vi "LabVIEW_MQTT_Toolkit_V2.vi"() -> ()   [LabVIEW 2021] (continued)
                  n338 = To Double Precision Float(number=w770) -> (double precision float=w775:dbl)
                  n339 = Number To Decimal String(number=w779) -> (decimal integer string=w778:string)  [unwired: 1 in]
                  n340 = Number To Fractional String(number=w777, precision (6)=i16 3 ("width (-)")) -> (F-format string=w781:string)  [unwired: 2 in]
                  n341 = Divide(x=w775, y=w771) -> (x/y=w776:dbl)
                  n342 = To Unsigned Quad Integer(1:w774) -> (0:w773:u64)
                  n343 = Build Array(w778, w781) -> (w780:string[])
                  n344 = call "Unix Time to Timestamp.vi"("Fractional Second"=w776, "Unix Time (s)"=w773) -> ("Timestamp"=w764:timestamp)  [unwired: 8 in, 1 out]
                  n345 = Format Date/Time String(seconds (now)=w764, UTC format=TRUE) -> (date/time string=w765:string)  [unwired: 1 in]
                  n346 = Scan From String(format string="%<%x %H:%M:%S%3u>T", input string=w765) -> (output 1=w766:timestamp)  [unwired: 3 in, 3 out]
                  n347 = To Double Precision Float(number=w766) -> (double precision float=w763:dbl)
                }
                n348 = Concatenate Strings(w724, "TimeStamp;MeasureCh_Y(g);", "\n") -> (w740:string)
                n349 = Concatenate Strings(w747, "_" ("string"), "streaming.csv") -> (w748:string)
                n350 = call <vilib>:"Get System Directory.vi"("system directory type"=w731) -> ("system directory"=w741:path)  [unwired: 10 in]
                n351 = Build Path(base path=w741, name or relative path="Logfile") -> (appended path=w742:path)
                n352 = call <vilib>:"Check if File or Folder Exists.vi"("path"=w742) -> ("file or folder exists?"=w743:bool, "dup path"=w744:path)  [unwired: 8 in, 1 out]
                n353 = case shown="False" w743 {
                  tunnel: w744 -> [w761 w762]
                  tunnel: [w760 w762] -> w745
                  frame False {
                    n354 = Create Folder(path (use dialog)=w761) -> (created path=w760:path)  [unwired: 2 in, 2 out]
                  }
                  frame True {
                  }
                }
                n355 = Build Path(base path=w745, name or relative path=w748) -> (appended path=w746:path)
                n356 = Open/Create/Replace File(file path (use dialog)=w746, operation (0:open)=T11."open or create") -> (refnum out=w739:refnum<file>, error out=w737:errorcluster)  [unwired: 4 in, 1 out]
                n357 = Write to Text File(file (use dialog)=w739, text=w740, error in=w737) -> (refnum out=w738:refnum<file>, error out=w736:errorcluster)  [unwired: 1 in, 1 out]
                n358 = Close File(refnum=w738, error in=w736) -> (path=w725:path)  [unwired: 1 out]
              }
              frame 5 {
                w790 = T14 2 items=["User Home"=0, "User Desktop"=1, "User Documents"=2, "User Application Data"=3, "User Preferences"=4, "User Temporary"=5, "Public Documents"=6, "Public Application Data"=7, "Public Preferences"=8, "Public Cache"=13, "System Core Libraries"=9, "System Installed Libraries"=10, "Application Files"=11, "Boot Volume Root"=12] ("system directory type")
                n359 = Decimate 1D Array(w820) -> (w816:dbl[], w817:dbl[])
                n360 = Search and Replace String(replace all?=TRUE ("replace all? (F)"), input string=w784, search string="/") -> (result string=w806:string)  [unwired: 5 in, 3 out]
                n361 = Concatenate Strings(w783, "TimeStamp;MeasureCh_Z(g);Ch_Y(g);", "\n") -> (w799:string)
                n362 = for {
                  tunnel: [w843] -> w818 mode=indexing
                  tunnel: w819 -> [w842] mode=indexing
                  tunnel: w816 -> [w840] mode=indexing
                  tunnel: w817 -> [w839] mode=indexing
                  tunnel: [w840] -> w815 mode=indexing
                  tunnel: [w839] -> w814 mode=indexing
                  tunnel: w813 -> [w834]
                  tunnel: w812 -> [w833]
                  tunnel: w811 -> [w832] mode=indexing
                  tunnel: w810 -> [w831]
                  tunnel: [w825] -> w809
                  tunnel: [w825] -> w808
                  n363 = Join Numbers(hi=w834, lo=w833) -> ((hi.lo)=w836:u32)
                  n364 = To Double Precision Float(number=w832) -> (double precision float=w837:dbl)
                  n365 = Number To Decimal String(number=w842) -> (decimal integer string=w841:string)  [unwired: 1 in]
                  n366 = Number To Fractional String(number=w840, precision (6)=i16 3 ("width (-)")) -> (F-format string=w845:string)  [unwired: 2 in]
                  n367 = Number To Fractional String(number=w839, precision (6)=i16 3 ("width (-)")) -> (F-format string=w844:string)  [unwired: 2 in]
                  n368 = Divide(x=w837, y=w831) -> (x/y=w838:dbl)
                  n369 = Build Array(w841, w845, w844) -> (w843:string[])
                  n370 = To Unsigned Quad Integer(1:w836) -> (0:w835:u64)
                  n371 = call "Unix Time to Timestamp.vi"("Fractional Second"=w838, "Unix Time (s)"=w835) -> ("Timestamp"=w826:timestamp)  [unwired: 8 in, 1 out]
                  n372 = Format Date/Time String(seconds (now)=w826, UTC format=TRUE) -> (date/time string=w827:string)  [unwired: 1 in]
                  n373 = Scan From String(format string="%<%x %H:%M:%S%3u>T", input string=w827) -> (output 1=w828:timestamp)  [unwired: 3 in, 3 out]
                  n374 = To Double Precision Float(number=w828) -> (double precision float=w825:dbl)
                }
                n375 = Concatenate Strings(w806, "_" ("string"), "streaming.csv") -> (w807:string)
                n376 = call <vilib>:"Get System Directory.vi"("system directory type"=w790) -> ("system directory"=w800:path)  [unwired: 10 in]
                n377 = Build Path(base path=w800, name or relative path="Logfile") -> (appended path=w801:path)
                n378 = call <vilib>:"Check if File or Folder Exists.vi"("path"=w801) -> ("file or folder exists?"=w802:bool, "dup path"=w803:path)  [unwired: 8 in, 1 out]
                n379 = case shown="False" w802 {
                  tunnel: w803 -> [w823 w824]
                  tunnel: [w822 w824] -> w804
                  frame False {
                    n380 = Create Folder(path (use dialog)=w823) -> (created path=w822:path)  [unwired: 2 in, 2 out]
                  }
                  frame True {
                  }
                }
                n381 = Build Path(base path=w804, name or relative path=w807) -> (appended path=w805:path)
                n382 = Open/Create/Replace File(file path (use dialog)=w805, operation (0:open)=T11."open or create") -> (refnum out=w798:refnum<file>, error out=w796:errorcluster)  [unwired: 4 in, 1 out]
                n383 = Write to Text File(file (use dialog)=w798, text=w799, error in=w796) -> (refnum out=w797:refnum<file>, error out=w795:errorcluster)  [unwired: 1 in, 1 out]
                n384 = Close File(refnum=w797, error in=w795) -> (path=w785:path)  [unwired: 1 out]
              }
              frame 6 {
                w855 = T14 2 items=["User Home"=0, "User Desktop"=1, "User Documents"=2, "User Application Data"=3, "User Preferences"=4, "User Temporary"=5, "Public Documents"=6, "Public Application Data"=7, "Public Preferences"=8, "Public Cache"=13, "System Core Libraries"=9, "System Installed Libraries"=10, "Application Files"=11, "Boot Volume Root"=12] ("system directory type")
                n385 = Decimate 1D Array(w885) -> (w883:dbl[], w882:dbl[])
                n386 = Search and Replace String(replace all?=TRUE ("replace all? (F)"), input string=w850, search string="/") -> (result string=w871:string)  [unwired: 5 in, 3 out]
                n387 = for {
                  tunnel: w883 -> [w905] mode=indexing
                  tunnel: w882 -> [w904] mode=indexing
                  tunnel: [w908] -> w881 mode=indexing
                  tunnel: w884 -> [w907] mode=indexing
                  tunnel: [w905] -> w880 mode=indexing
                  tunnel: [w904] -> w879 mode=indexing
                  tunnel: w878 -> [w899]
                  tunnel: w877 -> [w898]
                  tunnel: w876 -> [w897] mode=indexing
                  tunnel: w875 -> [w896]
                  tunnel: [w890] -> w874
                  tunnel: [w890] -> w873
                  n388 = Join Numbers(hi=w899, lo=w898) -> ((hi.lo)=w901:u32)
                  n389 = To Double Precision Float(number=w897) -> (double precision float=w902:dbl)
                  n390 = Number To Decimal String(number=w907) -> (decimal integer string=w906:string)  [unwired: 1 in]
                  n391 = Number To Fractional String(number=w905, precision (6)=i16 3 ("width (-)")) -> (F-format string=w910:string)  [unwired: 2 in]
                  n392 = Number To Fractional String(number=w904, precision (6)=i16 3 ("width (-)")) -> (F-format string=w909:string)  [unwired: 2 in]
                  n393 = Divide(x=w902, y=w896) -> (x/y=w903:dbl)
                  n394 = Build Array(w906, w910, w909) -> (w908:string[])
                  n395 = To Unsigned Quad Integer(1:w901) -> (0:w900:u64)
                  n396 = call "Unix Time to Timestamp.vi"("Fractional Second"=w903, "Unix Time (s)"=w900) -> ("Timestamp"=w891:timestamp)  [unwired: 8 in, 1 out]
                  n397 = Format Date/Time String(seconds (now)=w891, UTC format=TRUE) -> (date/time string=w892:string)  [unwired: 1 in]
                  n398 = Scan From String(format string="%<%x %H:%M:%S%3u>T", input string=w892) -> (output 1=w893:timestamp)  [unwired: 3 in, 3 out]
                  n399 = To Double Precision Float(number=w893) -> (double precision float=w890:dbl)
                }
                n400 = Concatenate Strings(w848, "TimeStamp;MeasureCh_X(g);Ch_Y(g);", "\n") -> (w864:string)
                n401 = Concatenate Strings(w871, "_" ("string"), "streaming.csv") -> (w872:string)
                n402 = call <vilib>:"Get System Directory.vi"("system directory type"=w855) -> ("system directory"=w865:path)  [unwired: 10 in]
                n403 = Build Path(base path=w865, name or relative path="Logfile") -> (appended path=w866:path)
                n404 = call <vilib>:"Check if File or Folder Exists.vi"("path"=w866) -> ("file or folder exists?"=w867:bool, "dup path"=w868:path)  [unwired: 8 in, 1 out]
                n405 = case shown="False" w867 {
                  tunnel: w868 -> [w888 w889]
                  tunnel: [w887 w889] -> w869
                  frame False {
                    n406 = Create Folder(path (use dialog)=w888) -> (created path=w887:path)  [unwired: 2 in, 2 out]
                  }
                  frame True {
                  }
                }
                n407 = Build Path(base path=w869, name or relative path=w872) -> (appended path=w870:path)
                n408 = Open/Create/Replace File(file path (use dialog)=w870, operation (0:open)=T11."open or create") -> (refnum out=w863:refnum<file>, error out=w861:errorcluster)  [unwired: 4 in, 1 out]
                n409 = Write to Text File(file (use dialog)=w863, text=w864, error in=w861) -> (refnum out=w862:refnum<file>, error out=w860:errorcluster)  [unwired: 1 in, 1 out]
                n410 = Close File(refnum=w862, error in=w860) -> (path=w849:path)  [unwired: 1 out]
              }
              frame 7 {
                w920 = T14 2 items=["User Home"=0, "User Desktop"=1, "User Documents"=2, "User Application Data"=3, "User Preferences"=4, "User Temporary"=5, "Public Documents"=6, "Public Application Data"=7, "Public Preferences"=8, "Public Cache"=13, "System Core Libraries"=9, "System Installed Libraries"=10, "Application Files"=11, "Boot Volume Root"=12] ("system directory type")
                n411 = Search and Replace String(replace all?=TRUE ("replace all? (F)"), input string=w915, search string="/") -> (result string=w936:string)  [unwired: 5 in, 3 out]
                n412 = Concatenate Strings(w913, "TimeStamp;MeasureCh_Z(g);Ch_X(g);Ch_Y(g);", "\n") -> (w929:string)
                n413 = Concatenate Strings(w936, "_" ("string"), "streaming.csv") -> (w937:string)
                n414 = call <vilib>:"Get System Directory.vi"("system directory type"=w920) -> ("system directory"=w930:path)  [unwired: 10 in]
                n415 = Decimate 1D Array(w953) -> (w952:dbl[], w951:dbl[], w950:dbl[])
                n416 = for {
                  tunnel: w952 -> [w974] mode=indexing
                  tunnel: w951 -> [w973] mode=indexing
                  tunnel: w950 -> [w972] mode=indexing
                  tunnel: [w977] -> w949 mode=indexing
                  tunnel: w948 -> [w976] mode=indexing
                  tunnel: [w974] -> w947 mode=indexing
                  tunnel: [w973] -> w946 mode=indexing
                  tunnel: [w972] -> w945 mode=indexing
                  tunnel: w944 -> [w967]
                  tunnel: w943 -> [w966]
                  tunnel: w942 -> [w965] mode=indexing
                  tunnel: w941 -> [w964]
                  tunnel: [w958] -> w940
                  tunnel: [w958] -> w939
                  tunnel: [w958] -> w938
                  n417 = Join Numbers(hi=w967, lo=w966) -> ((hi.lo)=w969:u32)
                  n418 = To Double Precision Float(number=w965) -> (double precision float=w970:dbl)
                  n419 = Number To Decimal String(number=w976) -> (decimal integer string=w975:string)  [unwired: 1 in]
                  n420 = Number To Fractional String(number=w974, precision (6)=i16 3 ("width (-)")) -> (F-format string=w981:string)  [unwired: 2 in]
                  n421 = Number To Fractional String(number=w973, precision (6)=i16 3 ("width (-)")) -> (F-format string=w980:string)  [unwired: 2 in]
                  n422 = Number To Fractional String(number=w972, precision (6)=i16 3 ("width (-)")) -> (F-format string=w978:string)  [unwired: 2 in]
                  n423 = Divide(x=w970, y=w964) -> (x/y=w971:dbl)
                  n424 = To Unsigned Quad Integer(1:w969) -> (0:w968:u64)
                  n425 = Build Array(w975, w981, w980, w978) -> (w977:string[])
                  n426 = call "Unix Time to Timestamp.vi"("Fractional Second"=w971, "Unix Time (s)"=w968) -> ("Timestamp"=w959:timestamp)  [unwired: 8 in, 1 out]
                  n427 = Format Date/Time String(seconds (now)=w959, UTC format=TRUE) -> (date/time string=w960:string)  [unwired: 1 in]
                  n428 = Scan From String(format string="%<%x %H:%M:%S%3u>T", input string=w960) -> (output 1=w961:timestamp)  [unwired: 3 in, 3 out]
                  n429 = To Double Precision Float(number=w961) -> (double precision float=w958:dbl)
                }
                n430 = Build Path(base path=w930, name or relative path="Logfile") -> (appended path=w931:path)
                n431 = call <vilib>:"Check if File or Folder Exists.vi"("path"=w931) -> ("file or folder exists?"=w932:bool, "dup path"=w933:path)  [unwired: 8 in, 1 out]
                n432 = case shown="False" w932 {
                  tunnel: w933 -> [w956 w957]
                  tunnel: [w955 w957] -> w934
                  frame False {
                    n433 = Create Folder(path (use dialog)=w956) -> (created path=w955:path)  [unwired: 2 in, 2 out]
                  }
                  frame True {
                  }
                }
                n434 = Build Path(base path=w934, name or relative path=w937) -> (appended path=w935:path)
                n435 = Open/Create/Replace File(file path (use dialog)=w935, operation (0:open)=T11."open or create") -> (refnum out=w928:refnum<file>, error out=w926:errorcluster)  [unwired: 4 in, 1 out]
                n436 = Write to Text File(file (use dialog)=w928, text=w929, error in=w926) -> (refnum out=w927:refnum<file>, error out=w925:errorcluster)  [unwired: 1 in, 1 out]
                n437 = Close File(refnum=w927, error in=w925) -> (path=w914:path)  [unwired: 1 out]
              }
              frame 8 {
                w991 = T14 2 items=["User Home"=0, "User Desktop"=1, "User Documents"=2, "User Application Data"=3, "User Preferences"=4, "User Temporary"=5, "Public Documents"=6, "Public Application Data"=7, "Public Preferences"=8, "Public Cache"=13, "System Core Libraries"=9, "System Installed Libraries"=10, "Application Files"=11, "Boot Volume Root"=12] ("system directory type")
                n438 = Decimate 1D Array(w1018) -> (w1015:dbl[])
                n439 = Search and Replace String(replace all?=TRUE ("replace all? (F)"), input string=w986, search string="/") -> (result string=w1007:string)  [unwired: 5 in, 3 out]
                n440 = Concatenate Strings(w984, "TimeStamp;Measure INC_X(Deg);", "\n") -> (w1000:string)
                n441 = for {
                  tunnel: [w1041] -> w1017 mode=indexing
                  tunnel: w1016 -> [w1038] mode=indexing
                  tunnel: w1015 -> [w1037] mode=indexing
                  tunnel: [w1037] -> w1014 mode=indexing
                  tunnel: w1013 -> [w1032]
                  tunnel: w1012 -> [w1031]
                  tunnel: w1011 -> [w1030] mode=indexing
                  tunnel: w1010 -> [w1029]
                  tunnel: [w1024] -> w1009
                  n442 = Join Numbers(hi=w1032, lo=w1031) -> ((hi.lo)=w1034:u32)
                  n443 = To Double Precision Float(number=w1030) -> (double precision float=w1035:dbl)
                  n444 = Number To Decimal String(number=w1038) -> (decimal integer string=w1040:string)  [unwired: 1 in]
                  n445 = Number To Fractional String(number=w1037, precision (6)=i16 3 ("width (-)")) -> (F-format string=w1039:string)  [unwired: 2 in]
                  n446 = Divide(x=w1035, y=w1029) -> (x/y=w1036:dbl)
                  n447 = To Unsigned Quad Integer(1:w1034) -> (0:w1033:u64)
                  n448 = Build Array(w1040, w1039) -> (w1041:string[])
                  n449 = call "Unix Time to Timestamp.vi"("Fractional Second"=w1036, "Unix Time (s)"=w1033) -> ("Timestamp"=w1023:timestamp)  [unwired: 8 in, 1 out]
                  n450 = Format Date/Time String(seconds (now)=w1023, UTC format=TRUE) -> (date/time string=w1025:string)  [unwired: 1 in]
                  n451 = Scan From String(format string="%<%x %H:%M:%S%3u>T", input string=w1025) -> (output 1=w1026:timestamp)  [unwired: 3 in, 3 out]
                  n452 = To Double Precision Float(number=w1026) -> (double precision float=w1024:dbl)
                }
                n453 = Concatenate Strings(w1007, "_" ("string"), "streaming.csv") -> (w1008:string)
                n454 = call <vilib>:"Get System Directory.vi"("system directory type"=w991) -> ("system directory"=w1001:path)  [unwired: 10 in]
                n455 = Build Path(base path=w1001, name or relative path="Logfile") -> (appended path=w1002:path)
                n456 = call <vilib>:"Check if File or Folder Exists.vi"("path"=w1002) -> ("file or folder exists?"=w1003:bool, "dup path"=w1004:path)  [unwired: 8 in, 1 out]
                n457 = case shown="False" w1003 {
                  tunnel: w1004 -> [w1021 w1022]
                  tunnel: [w1020 w1022] -> w1005
                  frame False {
                    n458 = Create Folder(path (use dialog)=w1021) -> (created path=w1020:path)  [unwired: 2 in, 2 out]
                  }
                  frame True {
                  }
                }
                n459 = Build Path(base path=w1005, name or relative path=w1008) -> (appended path=w1006:path)
                n460 = Open/Create/Replace File(file path (use dialog)=w1006, operation (0:open)=T11."open or create") -> (refnum out=w999:refnum<file>, error out=w997:errorcluster)  [unwired: 4 in, 1 out]
                n461 = Write to Text File(file (use dialog)=w999, text=w1000, error in=w997) -> (refnum out=w998:refnum<file>, error out=w996:errorcluster)  [unwired: 1 in, 1 out]
                n462 = Close File(refnum=w998, error in=w996) -> (path=w985:path)  [unwired: 1 out]
              }
              frame 9 {
                w1050 = T14 2 items=["User Home"=0, "User Desktop"=1, "User Documents"=2, "User Application Data"=3, "User Preferences"=4, "User Temporary"=5, "Public Documents"=6, "Public Application Data"=7, "Public Preferences"=8, "Public Cache"=13, "System Core Libraries"=9, "System Installed Libraries"=10, "Application Files"=11, "Boot Volume Root"=12] ("system directory type")
                n463 = Decimate 1D Array(w1080) -> (w1076:dbl[], w1079:dbl[])
                n464 = Search and Replace String(replace all?=TRUE ("replace all? (F)"), input string=w1045, search string="/") -> (result string=w1066:string)  [unwired: 5 in, 3 out]
                n465 = for {
                  tunnel: [w1103] -> w1077 mode=indexing
                  tunnel: w1076 -> [w1100] mode=indexing
                  tunnel: w1079 -> [w1099] mode=indexing
                  tunnel: w1078 -> [w1101] mode=indexing
                  tunnel: [w1100] -> w1075 mode=indexing
                  tunnel: [w1099] -> w1074 mode=indexing
                  tunnel: w1073 -> [w1094]
                  tunnel: w1072 -> [w1093]
                  tunnel: w1071 -> [w1092] mode=indexing
                  tunnel: w1070 -> [w1091]
                  tunnel: [w1085] -> w1068
                  tunnel: [w1085] -> w1069
                  n466 = Join Numbers(hi=w1094, lo=w1093) -> ((hi.lo)=w1096:u32)
                  n467 = To Double Precision Float(number=w1092) -> (double precision float=w1097:dbl)
                  n468 = Number To Decimal String(number=w1101) -> (decimal integer string=w1102:string)  [unwired: 1 in]
                  n469 = Number To Fractional String(number=w1100, precision (6)=i16 3 ("width (-)")) -> (F-format string=w1105:string)  [unwired: 2 in]
                  n470 = Number To Fractional String(number=w1099, precision (6)=i16 3 ("width (-)")) -> (F-format string=w1104:string)  [unwired: 2 in]
                  n471 = Divide(x=w1097, y=w1091) -> (x/y=w1098:dbl)
                  n472 = Build Array(w1102, w1105, w1104) -> (w1103:string[])
                  n473 = To Unsigned Quad Integer(1:w1096) -> (0:w1095:u64)
                  n474 = call "Unix Time to Timestamp.vi"("Fractional Second"=w1098, "Unix Time (s)"=w1095) -> ("Timestamp"=w1086:timestamp)  [unwired: 8 in, 1 out]
                  n475 = Format Date/Time String(seconds (now)=w1086, UTC format=TRUE) -> (date/time string=w1090:string)  [unwired: 1 in]
                  n476 = Scan From String(format string="%<%x %H:%M:%S%3u>T", input string=w1090) -> (output 1=w1089:timestamp)  [unwired: 3 in, 3 out]
                  n477 = To Double Precision Float(number=w1089) -> (double precision float=w1085:dbl)
                }
                n478 = Concatenate Strings(w1043, "TimeStamp;Measure Ch_Z(g);INC_X(Deg);", "\n") -> (w1059:string)
                n479 = Concatenate Strings(w1066, "_" ("string"), "streaming.csv") -> (w1067:string)
                n480 = call <vilib>:"Get System Directory.vi"("system directory type"=w1050) -> ("system directory"=w1060:path)  [unwired: 10 in]
                n481 = Build Path(base path=w1060, name or relative path="Logfile") -> (appended path=w1061:path)
                n482 = call <vilib>:"Check if File or Folder Exists.vi"("path"=w1061) -> ("file or folder exists?"=w1062:bool, "dup path"=w1063:path)  [unwired: 8 in, 1 out]
                n483 = case shown="False" w1062 {
                  tunnel: w1063 -> [w1083 w1084]
                  tunnel: [w1082 w1084] -> w1064
                  frame False {
                    n484 = Create Folder(path (use dialog)=w1083) -> (created path=w1082:path)  [unwired: 2 in, 2 out]
                  }
                  frame True {
                  }
                }
                n485 = Build Path(base path=w1064, name or relative path=w1067) -> (appended path=w1065:path)
                n486 = Open/Create/Replace File(file path (use dialog)=w1065, operation (0:open)=T11."open or create") -> (refnum out=w1058:refnum<file>, error out=w1056:errorcluster)  [unwired: 4 in, 1 out]
                n487 = Write to Text File(file (use dialog)=w1058, text=w1059, error in=w1056) -> (refnum out=w1057:refnum<file>, error out=w1055:errorcluster)  [unwired: 1 in, 1 out]
                n488 = Close File(refnum=w1057, error in=w1055) -> (path=w1044:path)  [unwired: 1 out]
              }
              frame 10 {
                w1115 = T14 2 items=["User Home"=0, "User Desktop"=1, "User Documents"=2, "User Application Data"=3, "User Preferences"=4, "User Temporary"=5, "Public Documents"=6, "Public Application Data"=7, "Public Preferences"=8, "Public Cache"=13, "System Core Libraries"=9, "System Installed Libraries"=10, "Application Files"=11, "Boot Volume Root"=12] ("system directory type")
                n489 = Decimate 1D Array(w1145) -> (w1142:dbl[], w1141:dbl[])
                n490 = Search and Replace String(replace all?=TRUE ("replace all? (F)"), input string=w1110, search string="/") -> (result string=w1131:string)  [unwired: 5 in, 3 out]
                n491 = for {
                  tunnel: [w1166] -> _ mode=indexing
                  tunnel: [w1170] -> w1143 mode=indexing
                  tunnel: w1144 -> [w1169] mode=indexing
                  tunnel: w1142 -> [w1166] mode=indexing
                  tunnel: w1141 -> [w1165] mode=indexing
                  tunnel: [w1166] -> w1140 mode=indexing
                  tunnel: [w1165] -> w1139 mode=indexing
                  tunnel: w1138 -> [w1160]
                  tunnel: w1137 -> [w1159]
                  tunnel: w1136 -> [w1158] mode=indexing
                  tunnel: w1135 -> [w1157]
                  tunnel: [w1150] -> w1134
                  tunnel: [w1150] -> w1133
                  n492 = Join Numbers(hi=w1160, lo=w1159) -> ((hi.lo)=w1162:u32)
                  n493 = To Double Precision Float(number=w1158) -> (double precision float=w1163:dbl)
                  n494 = Number To Decimal String(number=w1169) -> (decimal integer string=w1168:string)  [unwired: 1 in]
                  n495 = Number To Fractional String(number=w1166, precision (6)=i16 3 ("width (-)")) -> (F-format string=w1171:string)  [unwired: 2 in]
                  n496 = Number To Fractional String(number=w1165, precision (6)=i16 3 ("width (-)")) -> (F-format string=w1167:string)  [unwired: 2 in]
                  n497 = Divide(x=w1163, y=w1157) -> (x/y=w1164:dbl)
                  n498 = Build Array(w1168, w1171, w1167) -> (w1170:string[])
                  n499 = To Unsigned Quad Integer(1:w1162) -> (0:w1161:u64)
                  n500 = call "Unix Time to Timestamp.vi"("Fractional Second"=w1164, "Unix Time (s)"=w1161) -> ("Timestamp"=w1151:timestamp)  [unwired: 8 in, 1 out]
                  n501 = Format Date/Time String(seconds (now)=w1151, UTC format=TRUE) -> (date/time string=w1152:string)  [unwired: 1 in]
                  n502 = Scan From String(format string="%<%x %H:%M:%S%3u>T", input string=w1152) -> (output 1=w1153:timestamp)  [unwired: 3 in, 3 out]
                  n503 = To Double Precision Float(number=w1153) -> (double precision float=w1150:dbl)
                }
                n504 = Concatenate Strings(w1108, "TimeStamp;Measure Ch_X(g);INC_X(Deg);", "\n") -> (w1124:string)
                n505 = Concatenate Strings(w1131, "_" ("string"), "streaming.csv") -> (w1132:string)
                n506 = call <vilib>:"Get System Directory.vi"("system directory type"=w1115) -> ("system directory"=w1125:path)  [unwired: 10 in]
                n507 = Build Path(base path=w1125, name or relative path="Logfile") -> (appended path=w1126:path)
                n508 = call <vilib>:"Check if File or Folder Exists.vi"("path"=w1126) -> ("file or folder exists?"=w1127:bool, "dup path"=w1128:path)  [unwired: 8 in, 1 out]
                n509 = case shown="False" w1127 {
                  tunnel: w1128 -> [w1148 w1149]
                  tunnel: [w1147 w1149] -> w1129
                  frame False {
                    n510 = Create Folder(path (use dialog)=w1148) -> (created path=w1147:path)  [unwired: 2 in, 2 out]
                  }
                  frame True {
                  }
                }
                n511 = Build Path(base path=w1129, name or relative path=w1132) -> (appended path=w1130:path)
                n512 = Open/Create/Replace File(file path (use dialog)=w1130, operation (0:open)=T11."open or create") -> (refnum out=w1123:refnum<file>, error out=w1121:errorcluster)  [unwired: 4 in, 1 out]
                n513 = Write to Text File(file (use dialog)=w1123, text=w1124, error in=w1121) -> (refnum out=w1122:refnum<file>, error out=w1120:errorcluster)  [unwired: 1 in, 1 out]
                n514 = Close File(refnum=w1122, error in=w1120) -> (path=w1109:path)  [unwired: 1 out]
              }
              frame 11 {
                w1180 = T14 2 items=["User Home"=0, "User Desktop"=1, "User Documents"=2, "User Application Data"=3, "User Preferences"=4, "User Temporary"=5, "Public Documents"=6, "Public Application Data"=7, "Public Preferences"=8, "Public Cache"=13, "System Core Libraries"=9, "System Installed Libraries"=10, "Application Files"=11, "Boot Volume Root"=12] ("system directory type")
                n515 = Search and Replace String(replace all?=TRUE ("replace all? (F)"), input string=w1175, search string="/") -> (result string=w1196:string)  [unwired: 5 in, 3 out]
                n516 = Concatenate Strings(w1173, "TimeStamp;Measure Ch_Z(g);Ch_X(g);INC_X(Deg);", "\n") -> (w1189:string)
                n517 = Concatenate Strings(w1196, "_" ("string"), "streaming.csv") -> (w1197:string)
                n518 = call <vilib>:"Get System Directory.vi"("system directory type"=w1180) -> ("system directory"=w1190:path)  [unwired: 10 in]
                n519 = Decimate 1D Array(w1213) -> (w1211:dbl[], w1210:dbl[], w1208:dbl[])
                n520 = for {
                  tunnel: [w1241] -> w1209 mode=indexing
                  tunnel: w1212 -> [w1238] mode=indexing
                  tunnel: w1211 -> [w1236] mode=indexing
                  tunnel: w1210 -> [w1235] mode=indexing
                  tunnel: w1208 -> [w1234] mode=indexing
                  tunnel: [w1236] -> w1207 mode=indexing
                  tunnel: [w1235] -> w1206 mode=indexing
                  tunnel: [w1234] -> w1205 mode=indexing
                  tunnel: w1204 -> [w1229]
                  tunnel: w1203 -> [w1228]
                  tunnel: w1202 -> [w1227] mode=indexing
                  tunnel: w1201 -> [w1226]
                  tunnel: [w1218] -> w1200
                  tunnel: [w1218] -> w1199
                  tunnel: [w1218] -> w1198
                  n521 = Join Numbers(hi=w1229, lo=w1228) -> ((hi.lo)=w1231:u32)
                  n522 = To Double Precision Float(number=w1227) -> (double precision float=w1232:dbl)
                  n523 = Number To Decimal String(number=w1238) -> (decimal integer string=w1240:string)  [unwired: 1 in]
                  n524 = Number To Fractional String(number=w1236, precision (6)=i16 3 ("width (-)")) -> (F-format string=w1242:string)  [unwired: 2 in]
                  n525 = Number To Fractional String(number=w1235, precision (6)=i16 3 ("width (-)")) -> (F-format string=w1239:string)  [unwired: 2 in]
                  n526 = Number To Fractional String(number=w1234, precision (6)=i16 3 ("width (-)")) -> (F-format string=w1237:string)  [unwired: 2 in]
                  n527 = Divide(x=w1232, y=w1226) -> (x/y=w1233:dbl)
                  n528 = To Unsigned Quad Integer(1:w1231) -> (0:w1230:u64)
                  n529 = Build Array(w1240, w1242, w1239, w1237) -> (w1241:string[])
                  n530 = call "Unix Time to Timestamp.vi"("Fractional Second"=w1233, "Unix Time (s)"=w1230) -> ("Timestamp"=w1219:timestamp)  [unwired: 8 in, 1 out]
                  n531 = Format Date/Time String(seconds (now)=w1219, UTC format=TRUE) -> (date/time string=w1220:string)  [unwired: 1 in]
                  n532 = Scan From String(format string="%<%x %H:%M:%S%3u>T", input string=w1220) -> (output 1=w1221:timestamp)  [unwired: 3 in, 3 out]
                  n533 = To Double Precision Float(number=w1221) -> (double precision float=w1218:dbl)
                }
                n534 = Build Path(base path=w1190, name or relative path="Logfile") -> (appended path=w1191:path)
                n535 = call <vilib>:"Check if File or Folder Exists.vi"("path"=w1191) -> ("file or folder exists?"=w1192:bool, "dup path"=w1193:path)  [unwired: 8 in, 1 out]
                n536 = case shown="False" w1192 {
                  tunnel: w1193 -> [w1216 w1217]
                  tunnel: [w1215 w1217] -> w1194
                  frame False {
                    n537 = Create Folder(path (use dialog)=w1216) -> (created path=w1215:path)  [unwired: 2 in, 2 out]
                  }
                  frame True {
                  }
                }
                n538 = Build Path(base path=w1194, name or relative path=w1197) -> (appended path=w1195:path)
                n539 = Open/Create/Replace File(file path (use dialog)=w1195, operation (0:open)=T11."open or create") -> (refnum out=w1188:refnum<file>, error out=w1186:errorcluster)  [unwired: 4 in, 1 out]
                n540 = Write to Text File(file (use dialog)=w1188, text=w1189, error in=w1186) -> (refnum out=w1187:refnum<file>, error out=w1185:errorcluster)  [unwired: 1 in, 1 out]
                n541 = Close File(refnum=w1187, error in=w1185) -> (path=w1174:path)  [unwired: 1 out]
              }
              frame 12 {
                w1251 = T14 2 items=["User Home"=0, "User Desktop"=1, "User Documents"=2, "User Application Data"=3, "User Preferences"=4, "User Temporary"=5, "Public Documents"=6, "Public Application Data"=7, "Public Preferences"=8, "Public Cache"=13, "System Core Libraries"=9, "System Installed Libraries"=10, "Application Files"=11, "Boot Volume Root"=12] ("system directory type")
                n542 = Decimate 1D Array(w1281) -> (w1279:dbl[], w1278:dbl[])
                n543 = Search and Replace String(replace all?=TRUE ("replace all? (F)"), input string=w1246, search string="/") -> (result string=w1267:string)  [unwired: 5 in, 3 out]
                n544 = for {
                  tunnel: [w1306] -> w1277 mode=indexing
                  tunnel: w1280 -> [w1303] mode=indexing
                  tunnel: w1279 -> [w1302] mode=indexing
                  tunnel: w1278 -> [w1301] mode=indexing
                  tunnel: [w1302] -> w1276 mode=indexing
                  tunnel: [w1301] -> w1275 mode=indexing
                  tunnel: w1274 -> [w1296]
                  tunnel: w1273 -> [w1295]
                  tunnel: w1272 -> [w1294] mode=indexing
                  tunnel: w1271 -> [w1293]
                  tunnel: [w1286] -> w1270
                  tunnel: [w1286] -> w1269
                  n545 = Join Numbers(hi=w1296, lo=w1295) -> ((hi.lo)=w1298:u32)
                  n546 = To Double Precision Float(number=w1294) -> (double precision float=w1299:dbl)
                  n547 = Number To Decimal String(number=w1303) -> (decimal integer string=w1305:string)  [unwired: 1 in]
                  n548 = Number To Fractional String(number=w1302, precision (6)=i16 3 ("width (-)")) -> (F-format string=w1307:string)  [unwired: 2 in]
                  n549 = Number To Fractional String(number=w1301, precision (6)=i16 3 ("width (-)")) -> (F-format string=w1304:string)  [unwired: 2 in]
                  n550 = Divide(x=w1299, y=w1293) -> (x/y=w1300:dbl)
                  n551 = Build Array(w1305, w1307, w1304) -> (w1306:string[])
                  n552 = To Unsigned Quad Integer(1:w1298) -> (0:w1297:u64)
                  n553 = call "Unix Time to Timestamp.vi"("Fractional Second"=w1300, "Unix Time (s)"=w1297) -> ("Timestamp"=w1287:timestamp)  [unwired: 8 in, 1 out]
                  n554 = Format Date/Time String(seconds (now)=w1287, UTC format=TRUE) -> (date/time string=w1288:string)  [unwired: 1 in]
                  n555 = Scan From String(format string="%<%x %H:%M:%S%3u>T", input string=w1288) -> (output 1=w1289:timestamp)  [unwired: 3 in, 3 out]
                  n556 = To Double Precision Float(number=w1289) -> (double precision float=w1286:dbl)
                }
                n557 = Concatenate Strings(w1244, "TimeStamp;Measure Ch_Y(g);INC_X(Deg);", "\n") -> (w1260:string)
                n558 = Concatenate Strings(w1267, "_" ("string"), "streaming.csv") -> (w1268:string)
                n559 = call <vilib>:"Get System Directory.vi"("system directory type"=w1251) -> ("system directory"=w1261:path)  [unwired: 10 in]
                n560 = Build Path(base path=w1261, name or relative path="Logfile") -> (appended path=w1262:path)
                n561 = call <vilib>:"Check if File or Folder Exists.vi"("path"=w1262) -> ("file or folder exists?"=w1263:bool, "dup path"=w1264:path)  [unwired: 8 in, 1 out]
                n562 = case shown="False" w1263 {
                  tunnel: w1264 -> [w1284 w1285]
                  tunnel: [w1283 w1285] -> w1265
                  frame False {
                    n563 = Create Folder(path (use dialog)=w1284) -> (created path=w1283:path)  [unwired: 2 in, 2 out]
                  }
                  frame True {
                  }
                }
                n564 = Build Path(base path=w1265, name or relative path=w1268) -> (appended path=w1266:path)
                n565 = Open/Create/Replace File(file path (use dialog)=w1266, operation (0:open)=T11."open or create") -> (refnum out=w1259:refnum<file>, error out=w1257:errorcluster)  [unwired: 4 in, 1 out]
                n566 = Write to Text File(file (use dialog)=w1259, text=w1260, error in=w1257) -> (refnum out=w1258:refnum<file>, error out=w1256:errorcluster)  [unwired: 1 in, 1 out]
                n567 = Close File(refnum=w1258, error in=w1256) -> (path=w1245:path)  [unwired: 1 out]
              }
              frame 13 {
                w1316 = T14 2 items=["User Home"=0, "User Desktop"=1, "User Documents"=2, "User Application Data"=3, "User Preferences"=4, "User Temporary"=5, "Public Documents"=6, "Public Application Data"=7, "Public Preferences"=8, "Public Cache"=13, "System Core Libraries"=9, "System Installed Libraries"=10, "Application Files"=11, "Boot Volume Root"=12] ("system directory type")
                n568 = Search and Replace String(replace all?=TRUE ("replace all? (F)"), input string=w1311, search string="/") -> (result string=w1332:string)  [unwired: 5 in, 3 out]
                n569 = Concatenate Strings(w1309, "TimeStamp;Measure Ch_Z(g);Ch_Y(g);INC_X(Deg)", "\n") -> (w1325:string)
                n570 = Concatenate Strings(w1332, "_" ("string"), "streaming.csv") -> (w1333:string)
                n571 = call <vilib>:"Get System Directory.vi"("system directory type"=w1316) -> ("system directory"=w1326:path)  [unwired: 10 in]
                n572 = Decimate 1D Array(w1349) -> (w1344:dbl[], w1347:dbl[], w1346:dbl[])
                n573 = for {
                  tunnel: [w1377] -> w1345 mode=indexing
                  tunnel: w1348 -> [w1373] mode=indexing
                  tunnel: w1344 -> [w1372] mode=indexing
                  tunnel: w1347 -> [w1371] mode=indexing
                  tunnel: w1346 -> [w1370] mode=indexing
                  tunnel: [w1372] -> w1343 mode=indexing
                  tunnel: [w1371] -> w1342 mode=indexing
                  tunnel: [w1370] -> w1341 mode=indexing
                  tunnel: w1340 -> [w1365]
                  tunnel: w1339 -> [w1364]
                  tunnel: w1338 -> [w1363] mode=indexing
                  tunnel: w1337 -> [w1362]
                  tunnel: [w1354] -> w1336
                  tunnel: [w1354] -> w1335
                  tunnel: [w1354] -> w1334
                  n574 = Join Numbers(hi=w1365, lo=w1364) -> ((hi.lo)=w1367:u32)
                  n575 = To Double Precision Float(number=w1363) -> (double precision float=w1368:dbl)
                  n576 = Number To Decimal String(number=w1373) -> (decimal integer string=w1376:string)  [unwired: 1 in]
                  n577 = Number To Fractional String(number=w1372, precision (6)=i16 3 ("width (-)")) -> (F-format string=w1378:string)  [unwired: 2 in]
                  n578 = Number To Fractional String(number=w1371, precision (6)=i16 3 ("width (-)")) -> (F-format string=w1375:string)  [unwired: 2 in]
                  n579 = Number To Fractional String(number=w1370, precision (6)=i16 3 ("width (-)")) -> (F-format string=w1374:string)  [unwired: 2 in]
                  n580 = Divide(x=w1368, y=w1362) -> (x/y=w1369:dbl)
                  n581 = To Unsigned Quad Integer(1:w1367) -> (0:w1366:u64)
                  n582 = Build Array(w1376, w1378, w1375, w1374) -> (w1377:string[])
                  n583 = call "Unix Time to Timestamp.vi"("Fractional Second"=w1369, "Unix Time (s)"=w1366) -> ("Timestamp"=w1355:timestamp)  [unwired: 8 in, 1 out]
                  n584 = Format Date/Time String(seconds (now)=w1355, UTC format=TRUE) -> (date/time string=w1356:string)  [unwired: 1 in]
                  n585 = Scan From String(format string="%<%x %H:%M:%S%3u>T", input string=w1356) -> (output 1=w1357:timestamp)  [unwired: 3 in, 3 out]
                  n586 = To Double Precision Float(number=w1357) -> (double precision float=w1354:dbl)
                }
                n587 = Build Path(base path=w1326, name or relative path="Logfile") -> (appended path=w1327:path)
                n588 = call <vilib>:"Check if File or Folder Exists.vi"("path"=w1327) -> ("file or folder exists?"=w1328:bool, "dup path"=w1329:path)  [unwired: 8 in, 1 out]
                n589 = case shown="False" w1328 {
                  tunnel: w1329 -> [w1352 w1353]
                  tunnel: [w1351 w1353] -> w1330
                  frame False {
                    n590 = Create Folder(path (use dialog)=w1352) -> (created path=w1351:path)  [unwired: 2 in, 2 out]
                  }
                  frame True {
                  }
                }
                n591 = Build Path(base path=w1330, name or relative path=w1333) -> (appended path=w1331:path)
                n592 = Open/Create/Replace File(file path (use dialog)=w1331, operation (0:open)=T11."open or create") -> (refnum out=w1324:refnum<file>, error out=w1322:errorcluster)  [unwired: 4 in, 1 out]
                n593 = Write to Text File(file (use dialog)=w1324, text=w1325, error in=w1322) -> (refnum out=w1323:refnum<file>, error out=w1321:errorcluster)  [unwired: 1 in, 1 out]
                n594 = Close File(refnum=w1323, error in=w1321) -> (path=w1310:path)  [unwired: 1 out]
              }
              frame 14 {
                w1387 = T14 2 items=["User Home"=0, "User Desktop"=1, "User Documents"=2, "User Application Data"=3, "User Preferences"=4, "User Temporary"=5, "Public Documents"=6, "Public Application Data"=7, "Public Preferences"=8, "Public Cache"=13, "System Core Libraries"=9, "System Installed Libraries"=10, "Application Files"=11, "Boot Volume Root"=12] ("system directory type")
                n595 = Search and Replace String(replace all?=TRUE ("replace all? (F)"), input string=w1382, search string="/") -> (result string=w1403:string)  [unwired: 5 in, 3 out]
                n596 = Concatenate Strings(w1380, "TimeStamp;Measure Ch_X(g);Ch_Y(g);INC_X(Deg)", "\n") -> (w1396:string)
                n597 = Concatenate Strings(w1403, "_" ("string"), "streaming.csv") -> (w1404:string)
                n598 = call <vilib>:"Get System Directory.vi"("system directory type"=w1387) -> ("system directory"=w1397:path)  [unwired: 10 in]
                n599 = Decimate 1D Array(w1420) -> (w1418:dbl[], w1417:dbl[], w1416:dbl[])
                n600 = for {
                  tunnel: [w1448] -> w1415 mode=indexing
                  tunnel: w1419 -> [w1444] mode=indexing
                  tunnel: w1418 -> [w1443] mode=indexing
                  tunnel: w1417 -> [w1442] mode=indexing
                  tunnel: w1416 -> [w1441] mode=indexing
                  tunnel: [w1443] -> w1414 mode=indexing
                  tunnel: [w1442] -> w1413 mode=indexing
                  tunnel: [w1441] -> w1412 mode=indexing
                  tunnel: w1411 -> [w1436]
                  tunnel: w1410 -> [w1435]
                  tunnel: w1409 -> [w1434] mode=indexing
                  tunnel: w1408 -> [w1433]
                  tunnel: [w1425] -> w1407
                  tunnel: [w1425] -> w1406
                  tunnel: [w1425] -> w1405
                  n601 = Join Numbers(hi=w1436, lo=w1435) -> ((hi.lo)=w1438:u32)
                  n602 = To Double Precision Float(number=w1434) -> (double precision float=w1439:dbl)
                  n603 = Number To Decimal String(number=w1444) -> (decimal integer string=w1447:string)  [unwired: 1 in]
                  n604 = Number To Fractional String(number=w1443, precision (6)=i16 3 ("width (-)")) -> (F-format string=w1449:string)  [unwired: 2 in]
                  n605 = Number To Fractional String(number=w1442, precision (6)=i16 3 ("width (-)")) -> (F-format string=w1446:string)  [unwired: 2 in]
                  n606 = Number To Fractional String(number=w1441, precision (6)=i16 3 ("width (-)")) -> (F-format string=w1445:string)  [unwired: 2 in]
                  n607 = Divide(x=w1439, y=w1433) -> (x/y=w1440:dbl)
                  n608 = To Unsigned Quad Integer(1:w1438) -> (0:w1437:u64)
                  n609 = Build Array(w1447, w1449, w1446, w1445) -> (w1448:string[])
                  n610 = call "Unix Time to Timestamp.vi"("Fractional Second"=w1440, "Unix Time (s)"=w1437) -> ("Timestamp"=w1426:timestamp)  [unwired: 8 in, 1 out]
                  n611 = Format Date/Time String(seconds (now)=w1426, UTC format=TRUE) -> (date/time string=w1427:string)  [unwired: 1 in]
                  n612 = Scan From String(format string="%<%x %H:%M:%S%3u>T", input string=w1427) -> (output 1=w1428:timestamp)  [unwired: 3 in, 3 out]
                  n613 = To Double Precision Float(number=w1428) -> (double precision float=w1425:dbl)
                }
                n614 = Build Path(base path=w1397, name or relative path="Logfile") -> (appended path=w1398:path)
                n615 = call <vilib>:"Check if File or Folder Exists.vi"("path"=w1398) -> ("file or folder exists?"=w1399:bool, "dup path"=w1400:path)  [unwired: 8 in, 1 out]
                n616 = case shown="False" w1399 {
                  tunnel: w1400 -> [w1423 w1424]
                  tunnel: [w1422 w1424] -> w1401
                  frame False {
                    n617 = Create Folder(path (use dialog)=w1423) -> (created path=w1422:path)  [unwired: 2 in, 2 out]
                  }
                  frame True {
                  }
                }
                n618 = Build Path(base path=w1401, name or relative path=w1404) -> (appended path=w1402:path)
                n619 = Open/Create/Replace File(file path (use dialog)=w1402, operation (0:open)=T11."open or create") -> (refnum out=w1395:refnum<file>, error out=w1393:errorcluster)  [unwired: 4 in, 1 out]
                n620 = Write to Text File(file (use dialog)=w1395, text=w1396, error in=w1393) -> (refnum out=w1394:refnum<file>, error out=w1392:errorcluster)  [unwired: 1 in, 1 out]
                n621 = Close File(refnum=w1394, error in=w1392) -> (path=w1381:path)  [unwired: 1 out]
              }
              frame 15 {
                w1458 = T14 2 items=["User Home"=0, "User Desktop"=1, "User Documents"=2, "User Application Data"=3, "User Preferences"=4, "User Temporary"=5, "Public Documents"=6, "Public Application Data"=7, "Public Preferences"=8, "Public Cache"=13, "System Core Libraries"=9, "System Installed Libraries"=10, "Application Files"=11, "Boot Volume Root"=12] ("system directory type")
                n622 = Search and Replace String(replace all?=TRUE ("replace all? (F)"), input string=w1453, search string="/") -> (result string=w1474:string)  [unwired: 5 in, 3 out]
                n623 = Concatenate Strings(w1451, "TimeStamp;MeasureCh_Z(g);Ch_X(g);Ch_Y(g);INC_X(Deg)", "\n") -> (w1467:string)
                n624 = Concatenate Strings(w1474, "_" ("string"), "streaming.csv") -> (w1475:string)
                n625 = call <vilib>:"Get System Directory.vi"("system directory type"=w1458) -> ("system directory"=w1468:path)  [unwired: 10 in]
                n626 = Decimate 1D Array(w1494) -> (w1492:dbl[], w1491:dbl[], w1490:dbl[], w1488:dbl[])
                n627 = for {
                  tunnel: [w1525] -> w1489 mode=indexing
                  tunnel: w1493 -> [w1520] mode=indexing
                  tunnel: w1492 -> [w1519] mode=indexing
                  tunnel: w1491 -> [w1518] mode=indexing
                  tunnel: w1490 -> [w1517] mode=indexing
                  tunnel: w1488 -> [w1516] mode=indexing
                  tunnel: [w1519] -> w1487 mode=indexing
                  tunnel: [w1518] -> w1486 mode=indexing
                  tunnel: [w1517] -> w1485 mode=indexing
                  tunnel: [w1516] -> w1484 mode=indexing
                  tunnel: w1483 -> [w1511]
                  tunnel: w1482 -> [w1510]
                  tunnel: w1481 -> [w1509] mode=indexing
                  tunnel: w1480 -> [w1508]
                  tunnel: [w1499] -> w1479
                  tunnel: [w1499] -> w1478
                  tunnel: [w1499] -> w1477
                  tunnel: [w1499] -> w1476
                  n628 = Join Numbers(hi=w1511, lo=w1510) -> ((hi.lo)=w1513:u32)
                  n629 = To Double Precision Float(number=w1509) -> (double precision float=w1514:dbl)
                  n630 = Number To Decimal String(number=w1520) -> (decimal integer string=w1524:string)  [unwired: 1 in]
                  n631 = Number To Fractional String(number=w1519, precision (6)=i16 3 ("width (-)")) -> (F-format string=w1526:string)  [unwired: 2 in]
                  n632 = Number To Fractional String(number=w1518, precision (6)=i16 3 ("width (-)")) -> (F-format string=w1523:string)  [unwired: 2 in]
                  n633 = Number To Fractional String(number=w1517, precision (6)=i16 3 ("width (-)")) -> (F-format string=w1522:string)  [unwired: 2 in]
                  n634 = Number To Fractional String(number=w1516, precision (6)=i16 3 ("width (-)")) -> (F-format string=w1521:string)  [unwired: 2 in]
                  n635 = Divide(x=w1514, y=w1508) -> (x/y=w1515:dbl)
                  n636 = To Unsigned Quad Integer(1:w1513) -> (0:w1512:u64)
                  n637 = Build Array(w1524, w1526, w1523, w1522, w1521) -> (w1525:string[])
                  n638 = call "Unix Time to Timestamp.vi"("Fractional Second"=w1515, "Unix Time (s)"=w1512) -> ("Timestamp"=w1500:timestamp)  [unwired: 8 in, 1 out]
                  n639 = Format Date/Time String(seconds (now)=w1500, UTC format=TRUE) -> (date/time string=w1504:string)  [unwired: 1 in]
                  n640 = Scan From String(format string="%<%x %H:%M:%S%3u>T", input string=w1504) -> (output 1=w1503:timestamp)  [unwired: 3 in, 3 out]
                  n641 = To Double Precision Float(number=w1503) -> (double precision float=w1499:dbl)
                }
                n642 = Build Path(base path=w1468, name or relative path="Logfile") -> (appended path=w1469:path)
                n643 = call <vilib>:"Check if File or Folder Exists.vi"("path"=w1469) -> ("file or folder exists?"=w1470:bool, "dup path"=w1471:path)  [unwired: 8 in, 1 out]
                n644 = case shown="False" w1470 {
                  tunnel: w1471 -> [w1497 w1498]
                  tunnel: [w1496 w1498] -> w1472
                  frame False {
                    n645 = Create Folder(path (use dialog)=w1497) -> (created path=w1496:path)  [unwired: 2 in, 2 out]
                  }
                  frame True {
                  }
                }
                n646 = Build Path(base path=w1472, name or relative path=w1475) -> (appended path=w1473:path)
                n647 = Open/Create/Replace File(file path (use dialog)=w1473, operation (0:open)=T11."open or create") -> (refnum out=w1466:refnum<file>, error out=w1464:errorcluster)  [unwired: 4 in, 1 out]
                n648 = Write to Text File(file (use dialog)=w1466, text=w1467, error in=w1464) -> (refnum out=w1465:refnum<file>, error out=w1463:errorcluster)  [unwired: 1 in, 1 out]
                n649 = Close File(refnum=w1465, error in=w1463) -> (path=w1452:path)  [unwired: 1 out]
              }
              frame 16 {
                w1535 = T14 2 items=["User Home"=0, "User Desktop"=1, "User Documents"=2, "User Application Data"=3, "User Preferences"=4, "User Temporary"=5, "Public Documents"=6, "Public Application Data"=7, "Public Preferences"=8, "Public Cache"=13, "System Core Libraries"=9, "System Installed Libraries"=10, "Application Files"=11, "Boot Volume Root"=12] ("system directory type")
                n650 = Decimate 1D Array(w1562) -> (w1560:dbl[])
                n651 = Search and Replace String(replace all?=TRUE ("replace all? (F)"), input string=w1530, search string="/") -> (result string=w1551:string)  [unwired: 5 in, 3 out]
                n652 = for {
                  tunnel: [w1584] -> w1559 mode=indexing
                  tunnel: w1561 -> [w1582] mode=indexing
                  tunnel: w1560 -> [w1581] mode=indexing
                  tunnel: [w1581] -> w1558 mode=indexing
                  tunnel: w1557 -> [w1576]
                  tunnel: w1556 -> [w1575]
                  tunnel: w1555 -> [w1574] mode=indexing
                  tunnel: w1554 -> [w1573]
                  tunnel: [w1567] -> w1553
                  n653 = Join Numbers(hi=w1576, lo=w1575) -> ((hi.lo)=w1578:u32)
                  n654 = To Double Precision Float(number=w1574) -> (double precision float=w1579:dbl)
                  n655 = Number To Decimal String(number=w1582) -> (decimal integer string=w1583:string)  [unwired: 1 in]
                  n656 = Number To Fractional String(number=w1581, precision (6)=i16 3 ("width (-)")) -> (F-format string=w1585:string)  [unwired: 2 in]
                  n657 = Divide(x=w1579, y=w1573) -> (x/y=w1580:dbl)
                  n658 = To Unsigned Quad Integer(1:w1578) -> (0:w1577:u64)
                  n659 = Build Array(w1583, w1585) -> (w1584:string[])
                  n660 = call "Unix Time to Timestamp.vi"("Fractional Second"=w1580, "Unix Time (s)"=w1577) -> ("Timestamp"=w1568:timestamp)  [unwired: 8 in, 1 out]
                  n661 = Format Date/Time String(seconds (now)=w1568, UTC format=TRUE) -> (date/time string=w1569:string)  [unwired: 1 in]
                  n662 = Scan From String(format string="%<%x %H:%M:%S%3u>T", input string=w1569) -> (output 1=w1570:timestamp)  [unwired: 3 in, 3 out]
                  n663 = To Double Precision Float(number=w1570) -> (double precision float=w1567:dbl)
                }
                n664 = Concatenate Strings(w1528, "TimeStamp;MeasureINC_Y(Deg)", "\n") -> (w1544:string)
                n665 = Concatenate Strings(w1551, "_" ("string"), "streaming.csv") -> (w1552:string)
                n666 = call <vilib>:"Get System Directory.vi"("system directory type"=w1535) -> ("system directory"=w1545:path)  [unwired: 10 in]
                n667 = Build Path(base path=w1545, name or relative path="Logfile") -> (appended path=w1546:path)
                n668 = call <vilib>:"Check if File or Folder Exists.vi"("path"=w1546) -> ("file or folder exists?"=w1547:bool, "dup path"=w1548:path)  [unwired: 8 in, 1 out]
                n669 = case shown="False" w1547 {
                  tunnel: w1548 -> [w1565 w1566]
                  tunnel: [w1564 w1566] -> w1549
                  frame False {
                    n670 = Create Folder(path (use dialog)=w1565) -> (created path=w1564:path)  [unwired: 2 in, 2 out]
                  }
                  frame True {
                  }
                }
                n671 = Build Path(base path=w1549, name or relative path=w1552) -> (appended path=w1550:path)
                n672 = Open/Create/Replace File(file path (use dialog)=w1550, operation (0:open)=T11."open or create") -> (refnum out=w1543:refnum<file>, error out=w1541:errorcluster)  [unwired: 4 in, 1 out]
                n673 = Write to Text File(file (use dialog)=w1543, text=w1544, error in=w1541) -> (refnum out=w1542:refnum<file>, error out=w1540:errorcluster)  [unwired: 1 in, 1 out]
                n674 = Close File(refnum=w1542, error in=w1540) -> (path=w1529:path)  [unwired: 1 out]
              }
              frame 17 {
                w1594 = T14 2 items=["User Home"=0, "User Desktop"=1, "User Documents"=2, "User Application Data"=3, "User Preferences"=4, "User Temporary"=5, "Public Documents"=6, "Public Application Data"=7, "Public Preferences"=8, "Public Cache"=13, "System Core Libraries"=9, "System Installed Libraries"=10, "Application Files"=11, "Boot Volume Root"=12] ("system directory type")
                n675 = Decimate 1D Array(w1624) -> (w1620:dbl[], w1622:dbl[])
                n676 = Search and Replace String(replace all?=TRUE ("replace all? (F)"), input string=w1589, search string="/") -> (result string=w1610:string)  [unwired: 5 in, 3 out]
                n677 = for {
                  tunnel: [w1649] -> w1621 mode=indexing
                  tunnel: w1623 -> [w1647] mode=indexing
                  tunnel: w1620 -> [w1644] mode=indexing
                  tunnel: w1622 -> [w1643] mode=indexing
                  tunnel: [w1644] -> w1619 mode=indexing
                  tunnel: [w1643] -> w1618 mode=indexing
                  tunnel: w1617 -> [w1638]
                  tunnel: w1616 -> [w1637]
                  tunnel: w1615 -> [w1636] mode=indexing
                  tunnel: w1614 -> [w1635]
                  tunnel: [w1629] -> w1613
                  tunnel: [w1629] -> w1612
                  n678 = Join Numbers(hi=w1638, lo=w1637) -> ((hi.lo)=w1640:u32)
                  n679 = To Double Precision Float(number=w1636) -> (double precision float=w1641:dbl)
                  n680 = Number To Decimal String(number=w1647) -> (decimal integer string=w1648:string)  [unwired: 1 in]
                  n681 = Number To Fractional String(number=w1644, precision (6)=i16 3 ("width (-)")) -> (F-format string=w1650:string)  [unwired: 2 in]
                  n682 = Number To Fractional String(number=w1643, precision (6)=i16 3 ("width (-)")) -> (F-format string=w1645:string)  [unwired: 2 in]
                  n683 = Divide(x=w1641, y=w1635) -> (x/y=w1642:dbl)
                  n684 = Build Array(w1648, w1650, w1645) -> (w1649:string[])
                  n685 = To Unsigned Quad Integer(1:w1640) -> (0:w1639:u64)
                  n686 = call "Unix Time to Timestamp.vi"("Fractional Second"=w1642, "Unix Time (s)"=w1639) -> ("Timestamp"=w1630:timestamp)  [unwired: 8 in, 1 out]
                  n687 = Format Date/Time String(seconds (now)=w1630, UTC format=TRUE) -> (date/time string=w1631:string)  [unwired: 1 in]
                  n688 = Scan From String(format string="%<%x %H:%M:%S%3u>T", input string=w1631) -> (output 1=w1632:timestamp)  [unwired: 3 in, 3 out]
                  n689 = To Double Precision Float(number=w1632) -> (double precision float=w1629:dbl)
                }
                n690 = Concatenate Strings(w1587, "TimeStamp;MeasureCh_Z(g);INC_Y(Deg)", "\n") -> (w1603:string)
                n691 = Concatenate Strings(w1610, "_" ("string"), "streaming.csv") -> (w1611:string)
                n692 = call <vilib>:"Get System Directory.vi"("system directory type"=w1594) -> ("system directory"=w1604:path)  [unwired: 10 in]
                n693 = Build Path(base path=w1604, name or relative path="Logfile") -> (appended path=w1605:path)
                n694 = call <vilib>:"Check if File or Folder Exists.vi"("path"=w1605) -> ("file or folder exists?"=w1606:bool, "dup path"=w1607:path)  [unwired: 8 in, 1 out]
                n695 = case shown="False" w1606 {
                  tunnel: w1607 -> [w1627 w1628]
                  tunnel: [w1626 w1628] -> w1608
                  frame False {
                    n696 = Create Folder(path (use dialog)=w1627) -> (created path=w1626:path)  [unwired: 2 in, 2 out]
                  }
                  frame True {
                  }
                }
                n697 = Build Path(base path=w1608, name or relative path=w1611) -> (appended path=w1609:path)
                n698 = Open/Create/Replace File(file path (use dialog)=w1609, operation (0:open)=T11."open or create") -> (refnum out=w1602:refnum<file>, error out=w1600:errorcluster)  [unwired: 4 in, 1 out]
                n699 = Write to Text File(file (use dialog)=w1602, text=w1603, error in=w1600) -> (refnum out=w1601:refnum<file>, error out=w1599:errorcluster)  [unwired: 1 in, 1 out]
                n700 = Close File(refnum=w1601, error in=w1599) -> (path=w1588:path)  [unwired: 1 out]
              }
              frame 18 {
                w1659 = T14 2 items=["User Home"=0, "User Desktop"=1, "User Documents"=2, "User Application Data"=3, "User Preferences"=4, "User Temporary"=5, "Public Documents"=6, "Public Application Data"=7, "Public Preferences"=8, "Public Cache"=13, "System Core Libraries"=9, "System Installed Libraries"=10, "Application Files"=11, "Boot Volume Root"=12] ("system directory type")
                n701 = Decimate 1D Array(w1688) -> (w1684:dbl[], w1686:dbl[])
                n702 = Search and Replace String(replace all?=TRUE ("replace all? (F)"), input string=w1653, search string="/") -> (result string=w1675:string)  [unwired: 5 in, 3 out]
                n703 = for {
                  tunnel: [w1713] -> w1685 mode=indexing
                  tunnel: w1687 -> [w1709] mode=indexing
                  tunnel: w1684 -> [w1708] mode=indexing
                  tunnel: w1686 -> [w1707] mode=indexing
                  tunnel: [w1708] -> w1683 mode=indexing
                  tunnel: [w1707] -> w1682 mode=indexing
                  tunnel: w1681 -> [w1702]
                  tunnel: w1680 -> [w1701]
                  tunnel: w1679 -> [w1700] mode=indexing
                  tunnel: w1678 -> [w1699]
                  tunnel: [w1694] -> w1677
                  n704 = Join Numbers(hi=w1702, lo=w1701) -> ((hi.lo)=w1704:u32)
                  n705 = To Double Precision Float(number=w1700) -> (double precision float=w1705:dbl)
                  n706 = Number To Decimal String(number=w1709) -> (decimal integer string=w1712:string)  [unwired: 1 in]
                  n707 = Number To Fractional String(number=w1708, precision (6)=i16 3 ("width (-)")) -> (F-format string=w1714:string)  [unwired: 2 in]
                  n708 = Number To Fractional String(number=w1707, precision (6)=i16 3 ("width (-)")) -> (F-format string=w1710:string)  [unwired: 2 in]
                  n709 = Divide(x=w1705, y=w1699) -> (x/y=w1706:dbl)
                  n710 = Build Array(w1712, w1714, w1710) -> (w1713:string[])
                  n711 = To Unsigned Quad Integer(1:w1704) -> (0:w1703:u64)
                  n712 = call "Unix Time to Timestamp.vi"("Fractional Second"=w1706, "Unix Time (s)"=w1703) -> ("Timestamp"=w1693:timestamp)  [unwired: 8 in, 1 out]
                  n713 = Format Date/Time String(seconds (now)=w1693, UTC format=TRUE) -> (date/time string=w1695:string)  [unwired: 1 in]
                  n714 = Scan From String(format string="%<%x %H:%M:%S%3u>T", input string=w1695) -> (output 1=w1696:timestamp)  [unwired: 3 in, 3 out]
                  n715 = To Double Precision Float(number=w1696) -> (double precision float=w1694:dbl)
                }
                n716 = Concatenate Strings(w1652, "TimeStamp;MeasureCh_X(g);INC_Y(Deg)", "\n") -> (w1668:string)
                n717 = Concatenate Strings(w1675, "_" ("string"), "streaming.csv") -> (w1676:string)
                n718 = call <vilib>:"Get System Directory.vi"("system directory type"=w1659) -> ("system directory"=w1669:path)  [unwired: 10 in]
                n719 = Build Path(base path=w1669, name or relative path="Logfile") -> (appended path=w1670:path)
                n720 = call <vilib>:"Check if File or Folder Exists.vi"("path"=w1670) -> ("file or folder exists?"=w1671:bool, "dup path"=w1672:path)  [unwired: 8 in, 1 out]
                n721 = case shown="False" w1671 {
                  tunnel: w1672 -> [w1691 w1692]
                  tunnel: [w1690 w1692] -> w1673
                  frame False {
                    n722 = Create Folder(path (use dialog)=w1691) -> (created path=w1690:path)  [unwired: 2 in, 2 out]
                  }
                  frame True {
                  }
                }
                n723 = Build Path(base path=w1673, name or relative path=w1676) -> (appended path=w1674:path)
